vi "GetAllAnalogInputVals.vi"(8 "error in (no error)":errorcluster, 11 "SerialPortRef":T1) -> (0 "error out":errorcluster, 2 "ADC input vals":u32[](array[numeric]), 3 "SerialPortRef 2":T1)   [LabVIEW 2015]
uses:
  <vilib>/Rock Robotics/WPI/SerialPort/WPI_SerialPortRef.ctl
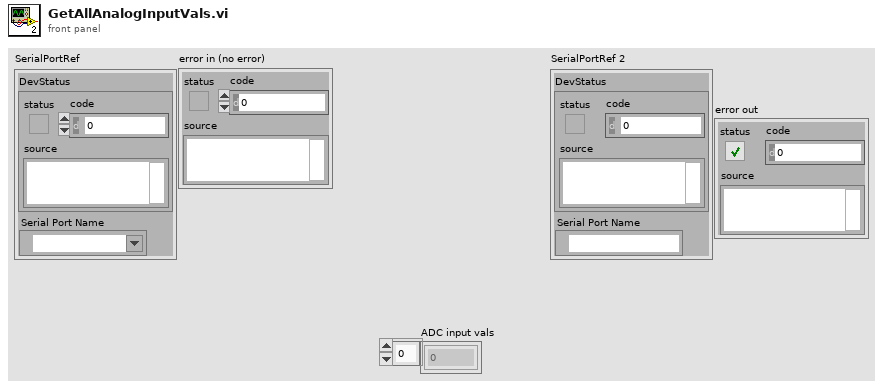
[diagram p1: front panel]
types:
  T1 = typedef "WPI_SerialPortRef.ctl" = cluster{"DevStatus":errorcluster, "Serial Port Name":refnum<visa-resource-name>}
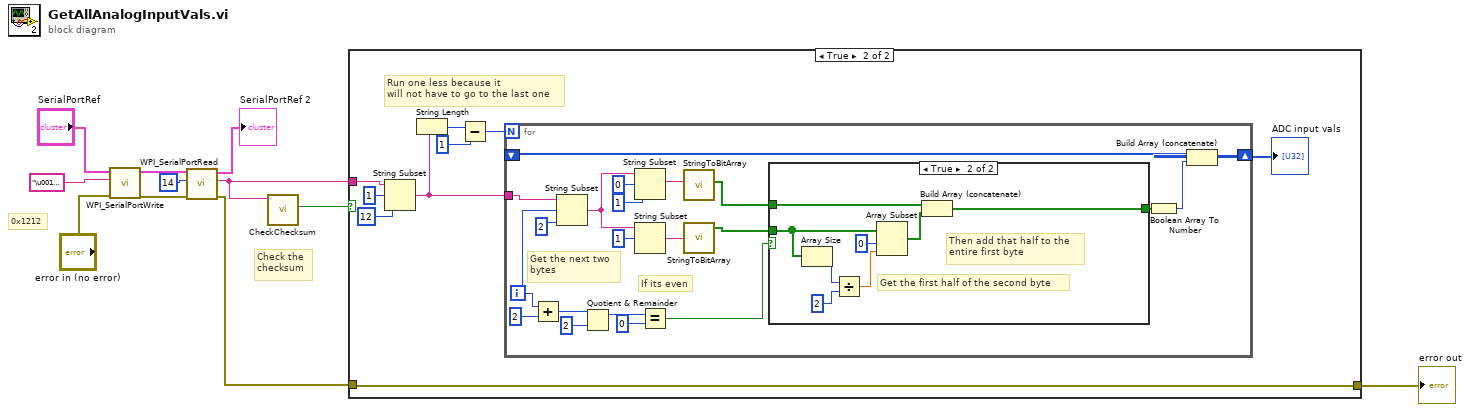
[diagram p0: block diagram]
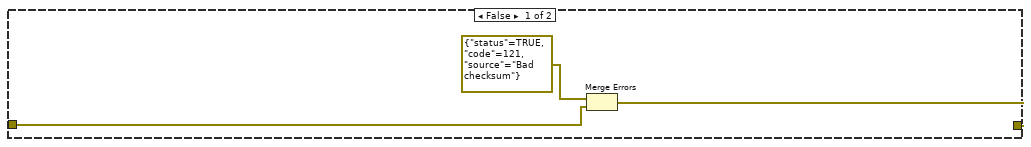
[diagram p2: hidden frame]
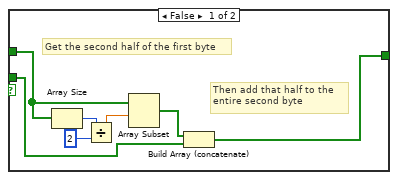
[diagram p3: hidden frame]
diagram:
  # "Check the\nchecksum"
  # "0x1212"
  n1 = call <vilib>:"WPI_SerialPortWrite.vi"("error in (no error)"="error in (no error)", "Buffer"="\u0012\u0012", "SerialPortRef"="SerialPortRef") -> ("error out"=w8:errorcluster, "SerialPortRef"=w9:T1)  [unwired: 6 in, 1 out]
  n2 = call <vilib>:"WPI_SerialPortRead.vi"("error in (no error)"=w8, "Num Bytes to Read"=u32 14, "SerialPortRef"=w9) -> ("error out"=w2:errorcluster, "Buffer"=w4:string, "SerialPortRef"=→"SerialPortRef 2":T1)  [unwired: 6 in]
  n3 = call "CheckChecksum.vi"("String"=w4) -> ("x = y?"=w3:bool)  [unwired: 10 in]
  n4 = case shown="True" w3 {
    tunnel: w4 -> [_ w16]
    tunnel: w2 -> [w13 w15]
    tunnel: [w12 w15] -> w1
    frame False {
      n5 = Merge Errors(errorcluster {"status"=TRUE, "code"=121, "source"="Bad checksum"} ("error in"), w13) -> (w12:errorcluster)
    }
    frame True {
      # "Run one less because it \nwill not have to go to the last one"
      n6 = String Subset(string=w16, offset (0)=1, length (rest)=12 ("length (rest)")) -> (substring=w21:string)
      n7 = String Length(string=w21) -> (length=w20:i32)
      n8 = Subtract(x=w20, y=1) -> (x-y=w18:i32)
      n9 = for {
        N: w18 -> [_]
        tunnel: w21 -> [w31]
        shift-right: [w32] -> w17
        shift-left: _ -> [w33]
        i -> [w30]
        # "If its even"
        # "Get the next two \nbytes"
        n10 = Add(x=w30, y=2) -> (x+y=w28:i32)
        n11 = String Subset(string=w31, offset (0)=w30, length (rest)=2 ("length (rest)")) -> (substring=w41:string)
        n12 = Quotient & Remainder(x=w28, y=2) -> (x-y*floor(x/y)=w26:i32)  [unwired: 1 out]
        n13 = String Subset(string=w41, offset (0)=0, length (rest)=1 ("length (rest)")) -> (substring=w38:string)
        n14 = String Subset(string=w41, offset (0)=1) -> (substring=w39:string)  [unwired: 1 in]
        n15 = Equal?(x=w26, y=0) -> (x = y?=w24:bool)
        n16 = call "StringToBitArray.vi"("string"=w38) -> ("Array"=w36:bool[])  [unwired: 10 in]
        n17 = call "StringToBitArray.vi"("string"=w39) -> ("Array"=w37:bool[])  [unwired: 10 in]
        n18 = case shown="True" w24 {
          tunnel: w37 -> [w47 w52]
          tunnel: w36 -> [w46 w55]
          tunnel: [w45 w53] -> w35
          frame False {
            # "Then add that half to the \nentire second byte"
            # "Get the second half of the first byte"
            n19 = Array Size(array=w46) -> (size(s)=w51:i32)
            n20 = Divide(x=w51, y=2) -> (x/y=w49:dbl)
            n21 = Array Subset(array=w46, index=w49) -> (w48:bool[])  [unwired: 1 in]
            n22 = Build Array (concatenate)(w48, w47) -> (w45:bool[])
          }
          frame True {
            # "Then add that half to the \nentire first byte"
            # "Get the first half of the second byte"
            n23 = Array Size(array=w52) -> (size(s)=w59:i32)
            n24 = Divide(x=w59, y=2) -> (x/y=w57:dbl)
            n25 = Array Subset(array=w52, index=0, length=w57) -> (w54:bool[])
            n26 = Build Array (concatenate)(w55, w54) -> (w53:bool[])
          }
        }
        n27 = Boolean Array To Number(Boolean array=w35) -> (number=w34:u32)
        n28 = Build Array (concatenate)(w33, w34) -> (w32:u32[])
      }
      "ADC input vals" <- w17
    }
  }
  "error out" <- w1
